vi "Format Message - Strip Tags.vi"(10 "opening tag":string, 11 "after open tag":string) -> (2 "format type":string, 3 "result string":string)   [LabVIEW 2021, in "Pop-Up.lvlib" / "Popup.lvclass"]
doc: "Remove the formatting tags from the string input - will strip off the first one so that string can continue to be processed for more tags.\n\n<b>Code Developed By:</b> +\nDaniel Coons +\nhttps://github.com/danielcoons/tsc-pop-up"
uses:
  Popup.lvclass
  Popup.lvclass/Popup.ctl
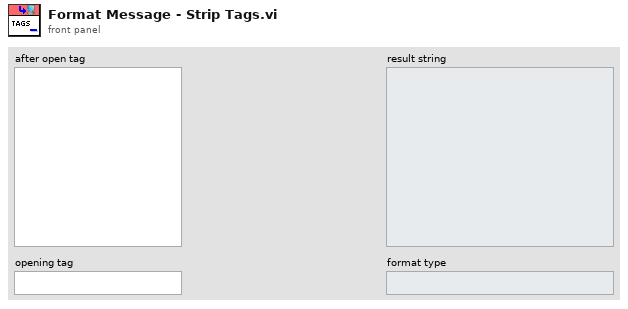
[diagram p1: front panel]
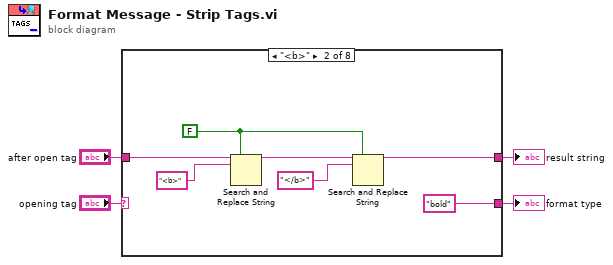
[diagram p0: block diagram]
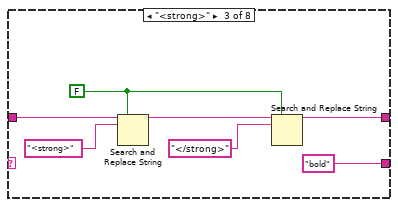
[diagram p3: hidden frame]
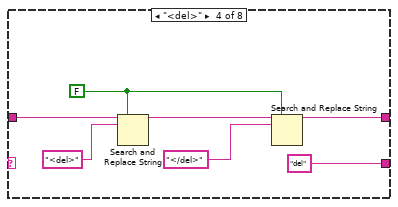
[diagram p4: hidden frame]
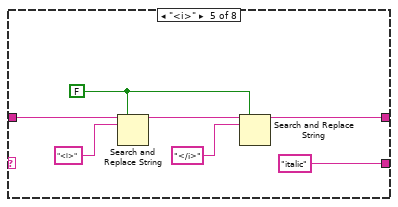
[diagram p5: hidden frame]
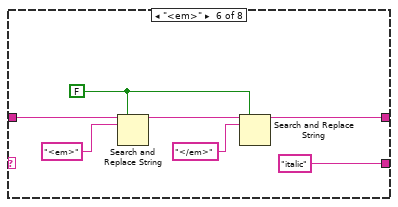
[diagram p6: hidden frame]
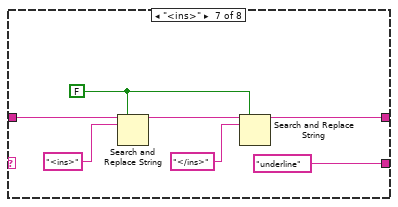
[diagram p7: hidden frame]
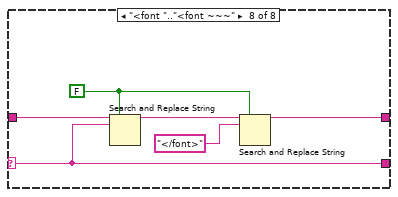
[diagram p8: hidden frame]
diagram:
  n1 = case shown="\"<b>\"" "opening tag" {
    selector: "opening tag" -> [_ _ _ _ _ _ _ w48]
    tunnel: "after open tag" -> [w5 w8 w15 w22 w29 w36 w43 w50]
    tunnel: [w5 w7 w13 w21 w27 w35 w42 w49] -> w1
    tunnel: [_ "bold" "bold" "del" "italic" "italic" "underline" w48] -> w2
    frame Default {
    }
    frame "<b>" {
      w11 = FALSE ("ignore case? (F)")
      n2 = Search and Replace String(replace all?=w11, input string=w8, search string="<b>") -> (result string=w12:string)  [unwired: 5 in, 3 out]
      n3 = Search and Replace String(replace all?=w11, input string=w12, search string="</b>") -> (result string=w7:string)  [unwired: 5 in, 3 out]
    }
    frame "<strong>" {
      w18 = FALSE ("ignore case? (F)")
      n4 = Search and Replace String(replace all?=w18, input string=w15, search string="<strong>") -> (result string=w19:string)  [unwired: 5 in, 3 out]
      n5 = Search and Replace String(replace all?=w18, input string=w19, search string="</strong>") -> (result string=w13:string)  [unwired: 5 in, 3 out]
    }
    frame "<del>" {
      w25 = FALSE ("ignore case? (F)")
      n6 = Search and Replace String(replace all?=w25, input string=w22, search string="<del>") -> (result string=w26:string)  [unwired: 5 in, 3 out]
      n7 = Search and Replace String(replace all?=w25, input string=w26, search string="</del>") -> (result string=w21:string)  [unwired: 5 in, 3 out]
    }
    frame "<i>" {
      w32 = FALSE ("ignore case? (F)")
      n8 = Search and Replace String(replace all?=w32, input string=w29, search string="<i>") -> (result string=w33:string)  [unwired: 5 in, 3 out]
      n9 = Search and Replace String(replace all?=w32, input string=w33, search string="</i>") -> (result string=w27:string)  [unwired: 5 in, 3 out]
    }
    frame "<em>" {
      w39 = FALSE ("ignore case? (F)")
      n10 = Search and Replace String(replace all?=w39, input string=w36, search string="<em>") -> (result string=w40:string)  [unwired: 5 in, 3 out]
      n11 = Search and Replace String(replace all?=w39, input string=w40, search string="</em>") -> (result string=w35:string)  [unwired: 5 in, 3 out]
    }
    frame "<ins>" {
      w46 = FALSE ("ignore case? (F)")
      n12 = Search and Replace String(replace all?=w46, input string=w43, search string="<ins>") -> (result string=w47:string)  [unwired: 5 in, 3 out]
      n13 = Search and Replace String(replace all?=w46, input string=w47, search string="</ins>") -> (result string=w42:string)  [unwired: 5 in, 3 out]
    }
    frame "<font ".."<font ~~~" {
      w52 = FALSE ("ignore case? (F)")
      n14 = Search and Replace String(replace all?=w52, input string=w50, search string=w48) -> (result string=w53:string)  [unwired: 5 in, 3 out]
      n15 = Search and Replace String(replace all?=w52, input string=w53, search string="</font>") -> (result string=w49:string)  [unwired: 5 in, 3 out]
    }
  }
  "format type" <- w2
  "result string" <- w1
